vi "_Raise Save File Security Check Starting.vi"(4 "WebView2.lvlib:WebView2 Control.lvclass":refnum<class "WebView2 Control.lvclass">, 5 "Event Data":cluster{"sender":refnum<k24>, "e":refnum<k24>}, 6 "Control Ref":refnum<k24>, 7 "Event Common Data":T1) -> ()   [LabVIEW 2025, in "WebView2.lvlib" / "WebView2 Control.lvclass"]
uses:
  WebView2 Control.lvclass
  WebView2 Control.lvclass/WebView2 Control.ctl
  E:/Labview/LV 2023/PPL/PPL Builder/Libs/LV-WebView2/Source/Libs/Microsoft.Web.WebView2.Core.dll
  Libs/Microsoft.Web.WebView2.Core.dll
  Save File Security Check Starting Event Data.ctl
  WebView2 Event Filter Interface/WebView2 Event Filter Interface.lvclass
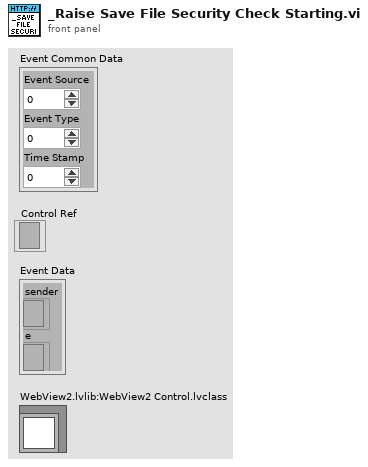
[diagram p1: front panel]
types:
  T1 = cluster{"Event Source":i32, "Event Type":u32, "Time Stamp":u32}
  T2 = typedef "WebView2.lvlib/WebView2 Control.lvclass/Save File Security Check Starting Event Data.ctl" = cluster{"DocumentOriginUri":string, "FileExtension":string, "FilePath":string}
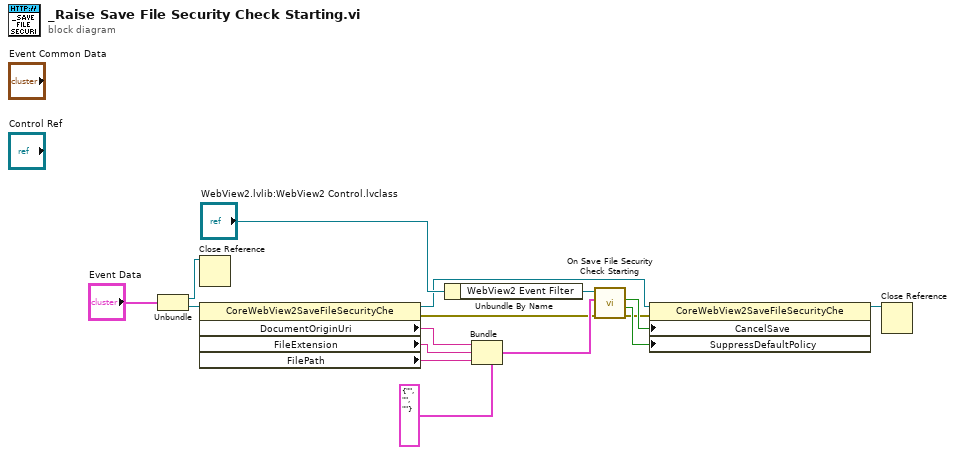
[diagram p0: block diagram]
diagram:
  n1 = Unbundle("Event Data") -> ("sender"=w15:refnum<k24>, "e"=w14:refnum<k24>)
  n2 = Close Reference(reference=w15) -> ()  [unwired: 1 in, 1 out]
  n3 = property class="CoreWebView2SaveFileSecurityChe"(reference=w14) -> (reference out=w6:refnum<k24>, error out=w3:errorcluster, "DocumentOriginUri"=w13:string, "FileExtension"=w12:string, "FilePath"=w11:string)  [unwired: 1 in]
  n4 = Unbundle By Name("WebView2.lvlib:WebView2 Control.lvclass") -> ("WebView2 Event Filter"=w8:refnum<class "WebView2 Event Filter Interface.lvclass">)
  n5 = Bundle(cluster=T2 {"DocumentOriginUri"="", "FileExtension"="", "FilePath"=""}, "DocumentOriginUri"=w13, "FileExtension"=w12, "FilePath"=w11) -> (w7:T2)
  n6 = call-dynamic "On Save File Security Check Starting.vi"("error in (no error)"=w3, "Data"=w7, "WebView2 Event Filter Interface in"=w8) -> ("error out"=w2:errorcluster, "SuppressDefaultPolicy"=w4:bool, "CancelSave"=w5:bool)  [unwired: 6 in]
  n7 = property class="CoreWebView2SaveFileSecurityChe"(reference=w6, error in=w2, "CancelSave"=w5, "SuppressDefaultPolicy"=w4) -> (reference out=w1:refnum<k24>)  [unwired: 1 out]
  n8 = Close Reference(reference=w1) -> ()  [unwired: 1 in, 1 out]
